vi "Shutdown Logging.vi"(8 "error in (no error)":errorcluster, 11 "Logging Thread in":refnum<class "Logging Thread.lvclass">) -> (0 "error out":errorcluster, 3 "Logging Thread out":refnum<class "Logging Thread.lvclass">)   [LabVIEW 2017, in "DSF Core.lvlib" / "Logging Thread.lvclass"]
uses:
  Logging Thread.lvclass
  Logging Thread.lvclass/Logging Thread.ctl
  Write Log File.vi
  Get Time.vi
  <vilib>/Utility/High Resolution Relative Seconds.vi
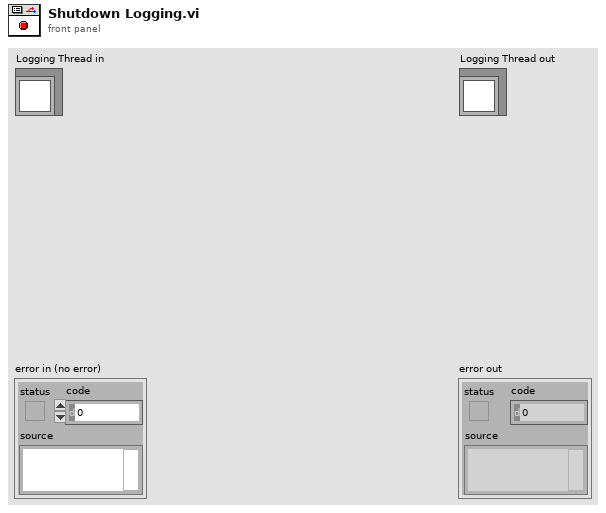
[diagram p1: front panel]
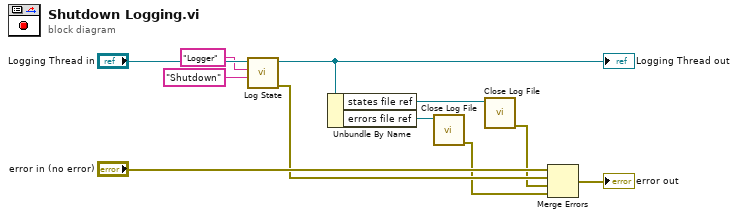
[diagram p0: block diagram]
diagram:
  n1 = call "Log State.vi"("line text"="Shutdown", "line tag"="Logger", "Logging Thread in"="Logging Thread in") -> ("error out"=w3:errorcluster, "Logging Thread out"=w6:refnum<class "Logging Thread.lvclass">)  [unwired: 7 in]
  "Logging Thread out" <- w6
  n2 = Unbundle By Name(w6) -> ("states file ref"=w10:refnum<file>, "errors file ref"=w11:refnum<file>)
  n3 = call "Close Log File.vi"("file refnum"=w11) -> ("error out"=w2:errorcluster)  [unwired: 10 in]
  n4 = call "Close Log File.vi"("file refnum"=w10) -> ("error out"=w1:errorcluster)  [unwired: 10 in]
  n5 = Merge Errors("error in (no error)", w3, w1, w2) -> (→"error out":errorcluster)
